vi "Talon Configuration.vi"   [LabVIEW 2013]
uses:
  <vilib>/Utility/file.llb/Read From Spreadsheet File (string).vi
types:
  T1 = typedef "WPI_MotorControlDeviceRef.ctl" = cluster{"DeviceStatus":errorcluster, "Type":enum16{"PWM", "CAN"}, "PWM":cluster{"Digital Module":T2, "PWM Channel":T3, "DeadBand":T4}, "CAN":cluster{"Device Number":u8, "Control Mode":T5, "Semaphore":T6, "Max Vout":dbl}, "Invert":bool, "TransformRef":T7, "InvTransformRef":T7}
  T2 = typedef "FPGA_TypedefDigitalModule.ctl" = enum16{"Digital Module 1", "Digital Module 2"}
  T3 = typedef "FPGA_DIOPWMChannel.ctl" = enum8{"PWM 1", "PWM 2", "PWM 3", "PWM 4", "PWM 5", "PWM 6", "PWM 7", "PWM 8", "PWM 9", "PWM 10", "Invalid"}
  T4 = typedef "WPI_PWMDeadband.ctl" = cluster{"Name":string, "maxPositivePwm":i32, "minPositivePwm":i32, "centerPwm":i32, "maxNegativePwm":i32, "minNegativePwm":i32, "angularRange":u16}
  T5 = typedef "WPI_CANJaguar_ControlMode.ctl" = enum8{"Percent VBus", "Current", "Speed", "Position", "Voltage"}
  T6 = typedef "Semaphore RefNum" = refnum<k1>
  T7 = typedef "WPI_PWMTransform_ConPane.ctl" = refnum<vi>
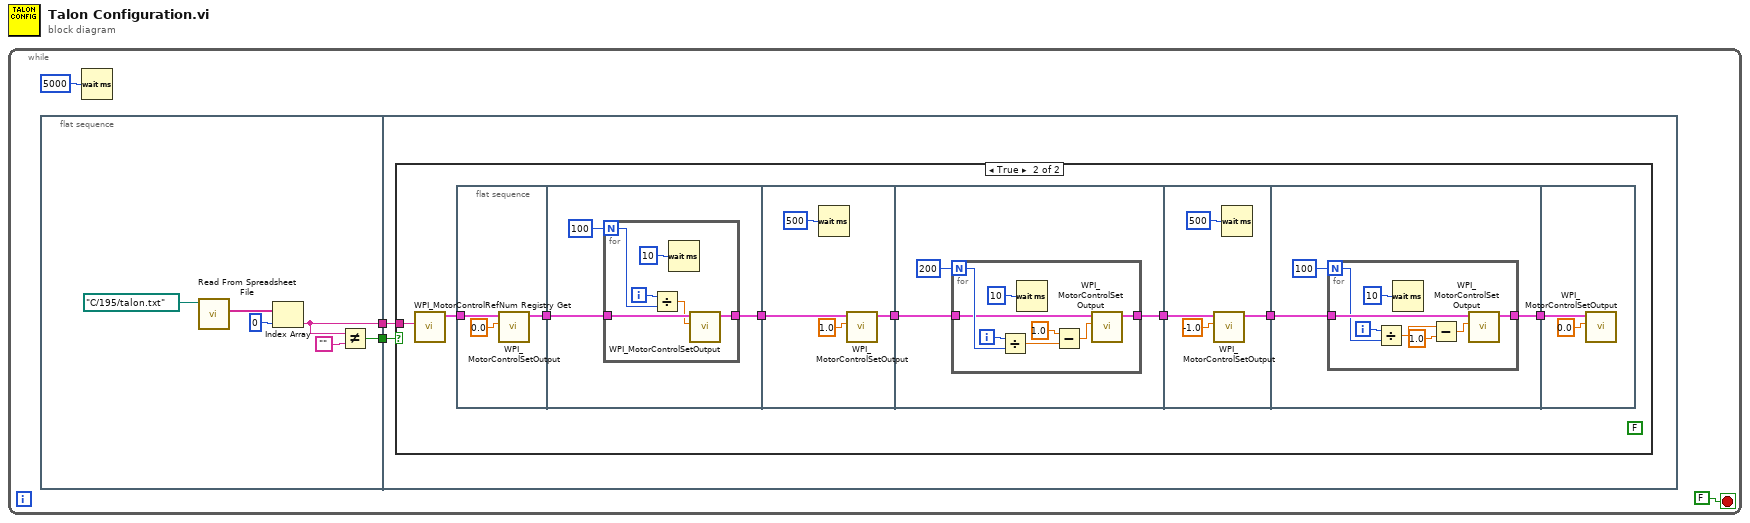
[diagram p0: block diagram]
diagram:
  n1 = while {
    stop <- FALSE stop-if-true
    n2 = flat-sequence {
      tunnel: [w7] -> w4
      tunnel: [w5] -> w3
      tunnel: w4 -> [w12]
      tunnel: w3 -> [w11]
      frame #0 {
        n3 = call-poly <vilib>:"Read From Spreadsheet File.vi"("file path (dialog if empty)"=path "C:/195/talon.txt" ("path")) -> ("first row"=w9:string[])  [unwired: 6 in, 4 out]
        n4 = Index Array(array=w9, index=0) -> (element=w5:string)
        n5 = Not Equal?(x=w5, y="") -> (x != y?=w7:bool)
      }
      frame #1 {
        n6 = case shown="True" w12 {
          tunnel: w11 -> [_ w20]
          frame False {
          }
          frame True {
            (unwired) FALSE
            n7 = call <vilib>:"WPI_MotorControlRefNum Registry Get.vi"("refnum name"=w20) -> ("MotorControlDevRef"=w19:T1)  [unwired: 9 in, 1 out]
            n8 = flat-sequence {
              tunnel: w19 -> [w23]
              tunnel: [w21] -> w18
              tunnel: w18 -> [w25]
              tunnel: [w24] -> w17
              tunnel: w17 -> [w36]
              tunnel: [w33] -> w16
              tunnel: w16 -> [w39]
              tunnel: [w37] -> w15
              tunnel: w15 -> [w49]
              tunnel: [w48] -> w14
              tunnel: w14 -> [w53]
              tunnel: [w52] -> w13
              tunnel: w13 -> [w63]
              frame #0 {
                n9 = call <vilib>:"WPI_MotorControlSetOutput.vi"("Output"=0.0, "MotorControlDevRef"=w23) -> ("MotorControlDevRef"=w21:T1)  [unwired: 7 in, 2 out]
              }
              frame #1 {
                n10 = for {
                  N: 100 -> [w28]
                  tunnel: w25 -> [w31]
                  tunnel: [w27] -> w24
                  i -> [w29]
                  n11 = Divide(x=w29, y=w28) -> (x/y=w30:dbl)
                  n12 = Wait (ms)(milliseconds to wait=u32 10) -> ()  [unwired: 1 out]
                  n13 = call <vilib>:"WPI_MotorControlSetOutput.vi"("Output"=w30, "MotorControlDevRef"=w31) -> ("MotorControlDevRef"=w27:T1)  [unwired: 7 in, 2 out]
                }
              }
              frame #2 {
                n14 = Wait (ms)(milliseconds to wait=u32 500) -> ()  [unwired: 1 out]
                n15 = call <vilib>:"WPI_MotorControlSetOutput.vi"("Output"=1.0, "MotorControlDevRef"=w36) -> ("MotorControlDevRef"=w33:T1)  [unwired: 7 in, 2 out]
              }
              frame #3 {
                n16 = for {
                  N: 200 -> [w45]
                  tunnel: w39 -> [w44]
                  tunnel: [w40] -> w37
                  i -> [w46]
                  n17 = Divide(x=w46, y=w45) -> (x/y=w43:dbl)
                  n18 = Wait (ms)(milliseconds to wait=u32 10) -> ()  [unwired: 1 out]
                  n19 = Subtract(x=1.0, y=w43) -> (x-y=w41:dbl)
                  n20 = call <vilib>:"WPI_MotorControlSetOutput.vi"("Output"=w41, "MotorControlDevRef"=w44) -> ("MotorControlDevRef"=w40:T1)  [unwired: 7 in, 2 out]
                }
              }
              frame #4 {
                n21 = call <vilib>:"WPI_MotorControlSetOutput.vi"("Output"=-1.0, "MotorControlDevRef"=w49) -> ("MotorControlDevRef"=w48:T1)  [unwired: 7 in, 2 out]
                n22 = Wait (ms)(milliseconds to wait=u32 500) -> ()  [unwired: 1 out]
              }
              frame #5 {
                n23 = for {
                  N: 100 -> [w59]
                  tunnel: w53 -> [w61]
                  tunnel: [w58] -> w52
                  i -> [w60]
                  n24 = Divide(x=w60, y=w59) -> (x/y=w57:dbl)
                  n25 = Wait (ms)(milliseconds to wait=u32 10) -> ()  [unwired: 1 out]
                  n26 = Subtract(x=w57, y=1.0) -> (x-y=w55:dbl)
                  n27 = call <vilib>:"WPI_MotorControlSetOutput.vi"("Output"=w55, "MotorControlDevRef"=w61) -> ("MotorControlDevRef"=w58:T1)  [unwired: 7 in, 2 out]
                }
              }
              frame #6 {
                n28 = call <vilib>:"WPI_MotorControlSetOutput.vi"("Output"=0.0, "MotorControlDevRef"=w63) -> ()  [unwired: 7 in, 3 out]
              }
            }
          }
        }
      }
    }
    n29 = Wait (ms)(milliseconds to wait=u32 5000) -> ()  [unwired: 1 out]
  }
